vi "ScaleImage.vi"(2 "Anti-aliasing (QT 6)":bool=TRUE, 3 "X scale":dbl=1.0 format="%.2f", 4 "Y scale":dbl=1.0 format="%.2f", 5 "Image in":T1 {"Dialogs" format="%.0b"}) -> (1 "Image Out":T1 {"Dialogs" format="%.0b"})   [LabVIEW 2024]
doc: "This VI will scale the X (horizontal) and Y (vertical) dimensions of an input image."
uses:
  <userlib>/ImageProcessing/QTLIB_2595_LV86/QT_Effect.ctl
  <userlib>/ImageProcessing/QTLIB_2595_LV86/QT_Private.ctl
  <userlib>/ImageProcessing/QTLIB_2595_LV86/QT_Image.ctl
panel:
  out "error out":errorcluster
  in  "error in (no error)":errorcluster
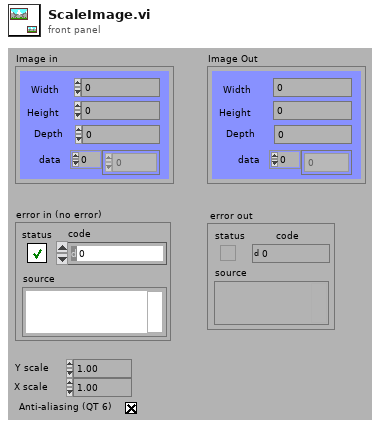
[diagram p1: front panel]
types:
  T1 = typedef "QT_Image.ctl" = cluster{"Width":i32, "Height":i32, "Depth":i32, "data":u8[], "Compressed data":u8[], "Color table":u32[], "Duration":i32, "Options":i32, "Timestamp":i32, "ID":i32, "Reserved":i32, "Dialogs":u32}
  T2 = typedef "QT_Private.ctl" = cluster{"reserved 1":i32, "reserved 2":i32, "reserved 3":i32, "reserved 4":i32}
  T3 = typedef "QT_Effect.ctl" = cluster{"Reserved":i32, "Matrix":dbl[]}
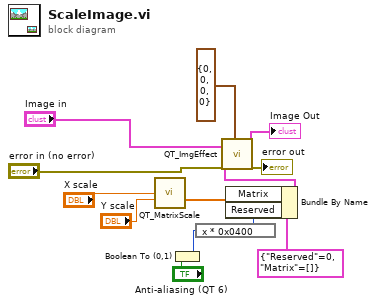
[diagram p0: block diagram]
diagram:
  n1 = call <userlib>:"QT_MatrixScale.vi"("X scale"="X scale", "Y scale"="Y scale") -> ("Out Matrix as Vector"=w11:dbl[])  [unwired: 2 in, 11 out]
  n2 = Boolean To (0,1)(Boolean="Anti-aliasing (QT 6)") -> (0, 1=w10:i16)
  n3 = expression code="x * 0x0400"(w10) -> (w8:i16)
  n4 = Bundle By Name(cluster=T3 {"Reserved"=0, "Matrix"=[]} ("Effect"), "Matrix"=w11, "Reserved"=w8) -> (w7:T3)
  n5 = call <userlib>:"QT_ImgEffect.vi"("Image In"="Image in", "Effect"=w7, "error in (no error)"="error in (no error)", "Private"=T2 {"reserved 1"=0, "reserved 2"=0, "reserved 3"=0, "reserved 4"=0}) -> ("Image Out"=→"Image Out":T1, "error out"=→"error out":errorcluster)  [unwired: 1 in, 13 out]
